vi "Stream WFM to Binary file (sgl).vi"(7 "Error In":errorcluster, 9 "Waveforms":waveform(dbl)[](array[waveform]), 10 "Refnum In":refnum<file>) -> (0 "Error Out":errorcluster, 3 "Refnum Out":refnum<file>)   [LabVIEW 2015]
uses:
  Processing/Trace (dbl).ctl
panel:
  in  "Trace":T1
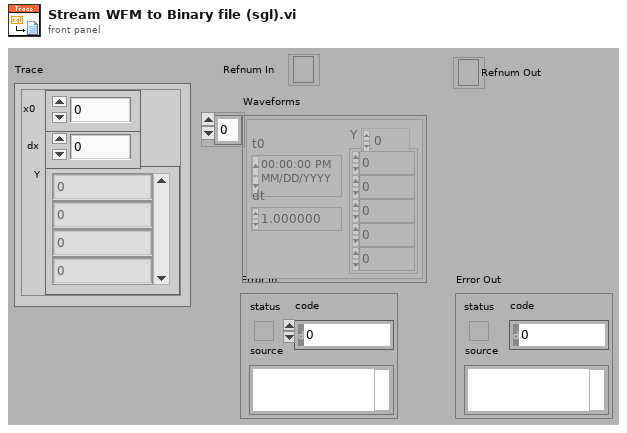
[diagram p1: front panel]
types:
  T1 = typedef "Trace (dbl).ctl" = cluster{"x0 ":dbl, "dx":dbl, "Y":dbl[]}
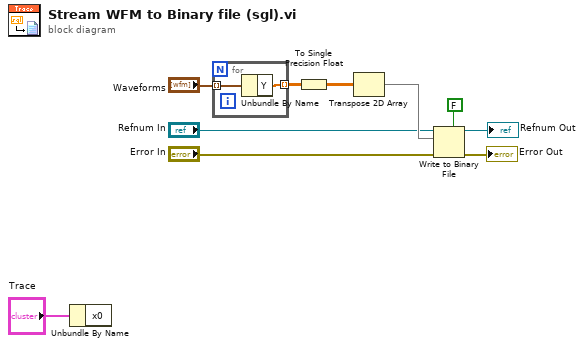
[diagram p0: block diagram]
diagram:
  n1 = Unbundle By Name("Trace") -> ()  [unwired: 1 out]
  n2 = for {
    tunnel: "Waveforms" -> [w12] mode=indexing
    tunnel: [w11] -> w5 mode=indexing
    n3 = Unbundle By Name(w12) -> ("Y"=w11:dbl[])
  }
  n4 = To Single Precision Float(number=w5) -> (single precision float=w9:sgl[][])
  n5 = Transpose 2D Array(2D array=w9) -> (transposed array=w10:sgl[][])
  n6 = Write to Binary File(file (use dialog)="Refnum In", data=w10, error in="Error In", 5:FALSE ("prepend array or string size? (T)")) -> (refnum out=→"Refnum Out":refnum<file>, error out=→"Error Out":errorcluster)  [unwired: 2 in, 1 out]
